vi "BL_LoadTechnique.vi"(0 "Potentiostat Galvanostat in":refnum<class "Potentiostat Galvanostat.lvclass">, 5 "Channel":u8 max=15, 7 "Technique File Name (.ecc)":string, 9 "Technique Parameters":T1 {"Parameter Type" items=["I32 (Long)", "BOOL (Boolean)", "SGL (Single Precision)"]}, 11 "error in (no error)":errorcluster, 12 "FirstTechnique":bool, 13 "LastTechnique":bool, 14 "DisplayParams":bool) -> (4 "Potentiostat Galvanostat out":refnum<class "Potentiostat Galvanostat.lvclass">, 6 "Channel":u8, 15 "error out":errorcluster)   [LabVIEW 2018, in "Potentiostat Galvanostat.lvclass"]
doc: "This function tests the communication speed between the library and the selected channel. \nNOTE: This function is for advanced user only."
uses:
  Potentiostat Galvanostat.lvclass
  Controls/Technique Parameters.ctl
  Controls/Technique Parameter.ctl
  Controls/Parameter Type.ctl
  Potentiostat Galvanostat.lvclass/Potentiostat Galvanostat.ctl
  BL_GetErrorMsg.vi
  <vilib>/Utility/error.llb/Error Cluster From Error Code.vi
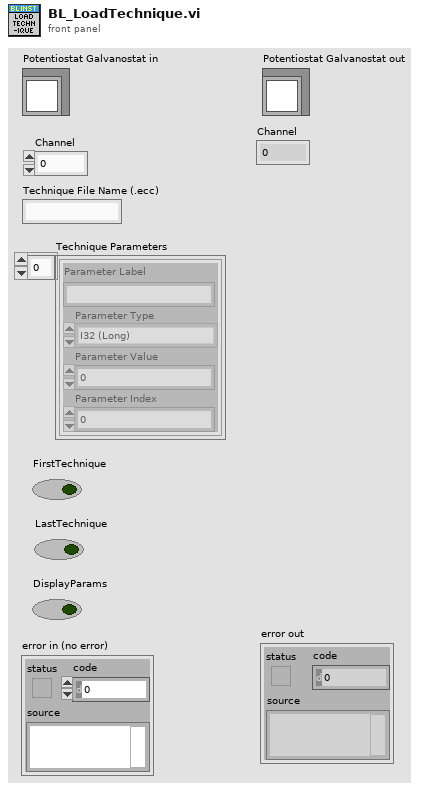
[diagram p1: front panel]
types:
  T1 = typedef "Potentiostat Galvanostat.lvclass/Technique Parameters.ctl" = T2[]
  T2 = typedef "Potentiostat Galvanostat.lvclass/Technique Parameter.ctl" = cluster{"Parameter Label":string, "Parameter Type":T3, "Parameter Value":i32, "Parameter Index":i32}
  T3 = typedef "Potentiostat Galvanostat.lvclass/Parameter Type.ctl" = i32
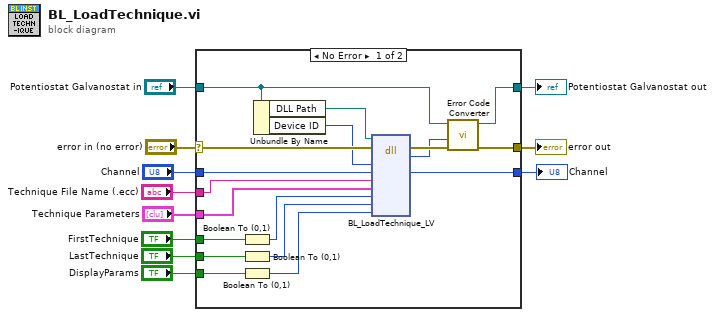
[diagram p0: block diagram]
diagram:
  n1 = case shown="No Error" "error in (no error)" {
    selector: "error in (no error)" -> [w26 w31]
    tunnel: [w29 w31] -> w10
    tunnel: [w27 w30] -> w8
    tunnel: "Potentiostat Galvanostat in" -> [w28 w30]
    tunnel: "Channel" -> [w21 _]
    tunnel: "Technique File Name (.ecc)" -> [w17 _]
    tunnel: "Technique Parameters" -> [w16 _]
    tunnel: "FirstTechnique" -> [w19 _]
    tunnel: "LastTechnique" -> [w18 _]
    tunnel: "DisplayParams" -> [w20 _]
    tunnel: [w12 _] -> w1
    frame No Error {
      n2 = Boolean To (0,1)(Boolean=w19) -> (0, 1=w15:i16)
      n3 = Boolean To (0,1)(Boolean=w18) -> (0, 1=w14:i16)
      n4 = Boolean To (0,1)(Boolean=w20) -> (0, 1=w13:i16)
      n5 = Unbundle By Name(w28) -> ("DLL Path"=w23:path, "Device ID"=w22:i32)
      n6 = dll-call lib="C:/Program Files (x86)/National Instruments/LabVIEW 2018/user.lib/EClib/EClib.*" fn="BL_LoadTechnique_LV"(path in=w23, error in=w26, "Device ID"=w22, "Channel"=w21, "Technique File Name(.ecc)"=w17, "Technique Parameters"=w16, "First Technique"=w15, "Last Technique"=w14, "Display Parameters?"=w13) -> (error out=w25:errorcluster, "Error Code"=w24:i32, "Channel"=w12:u8)  [unwired: 7 in, 1 out]
      n7 = call "Error Code Converter.vi"("error in (no error)"=w25, "Error Code"=w24, "Potentiostat Galvanostat in"=w28) -> ("error out"=w29:errorcluster, "Potentiostat Galvanostat out"=w27:refnum<class "Potentiostat Galvanostat.lvclass">)  [unwired: 7 in]
    }
    frame Error {
    }
  }
  "error out" <- w10
  "Potentiostat Galvanostat out" <- w8
  "Channel" <- w1
